vi "Area Scoring Ball.vi"(10 "Convex Hull Area":dbl, 11 "Area":dbl) -> (3 "Score":dbl)   [LabVIEW 2025]
doc: "Calculate a score based on area and convex hull area. Convex hull area fills holes and convex areas of the shape. It is equivalent to putting a rubber band around the shape and computing the area enclosed by the band."
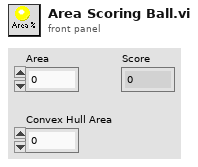
[diagram p1: front panel]
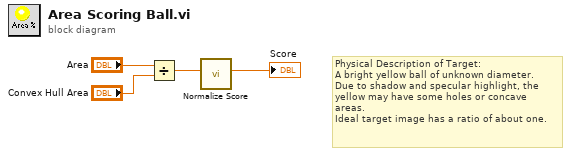
[diagram p0: block diagram]
diagram:
  # "Physical Description of Target:\nA bright yellow ball of unknown diameter.\nDue to shadow and specular highlight, the\nyellow may have some holes or concave \nareas.\nIdeal target image has a ratio of about one."
  n1 = Divide(x="Area", y="Convex Hull Area") -> (x/y=w1:dbl)
  n2 = call "Normalize Score.vi"("Value"=w1) -> ("Score"=→"Score":dbl)  [unwired: 10 in]
